vi "VelocityFix.vi"(9 "Tolerance":dbl=1e-05, 10 "Smooth Vel":dbl[][](array[numeric]), 11 "Orig Vel":dbl[][](array[numeric])) -> (3 "Fixed Vel":dbl[][](array[numeric]))   [LabVIEW 2016]
panel:
  out "Array":dbl[](array[numeric])
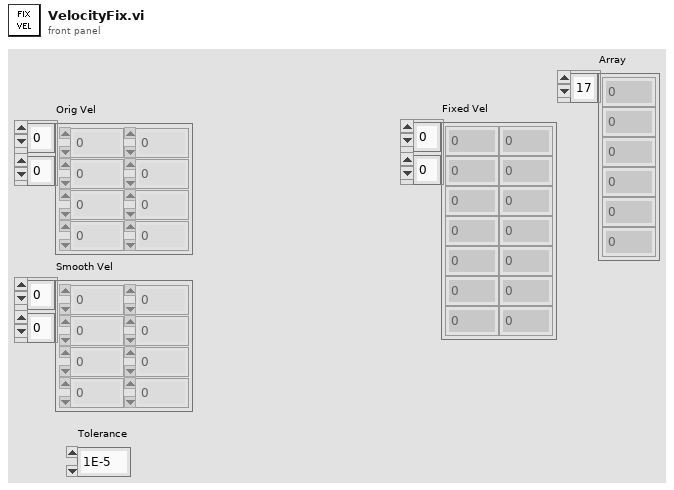
[diagram p1: front panel]
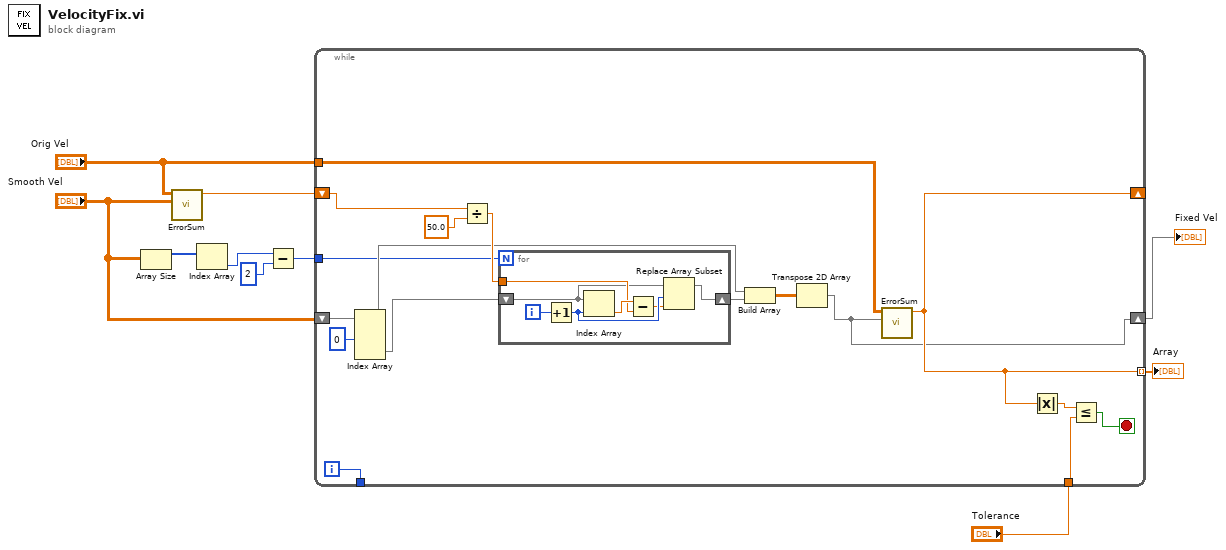
[diagram p0: block diagram]
diagram:
  n1 = Array Size(array="Smooth Vel") -> (size(s)=w3:i32[])
  n2 = call "ErrorSum.vi"("Smooth Vel"="Smooth Vel", "Orig Vel"="Orig Vel") -> ("Difference"=w9:dbl)  [unwired: 9 in]
  n3 = Index Array(array=w3) -> (element=w2:i32)  [unwired: 1 in]
  n4 = Subtract(x=w2, y=2) -> (x-y=w6:i32)
  n5 = while {
    tunnel: "Tolerance" -> [w26]
    tunnel: w6 -> [w12]
    tunnel: "Orig Vel" -> [w21]
    shift-right: [w17] -> _
    shift-left: w9 -> [w19]
    tunnel: [w18] -> _
    tunnel: [w17] -> w5 mode=indexing
    shift-right: [w11] -> w7
    shift-left: "Smooth Vel" -> [w15]
    i -> [w18]
    stop <- w27 stop-if-true
    n6 = Index Array(array=w15, index (col) #1=0 ("disabled index (col)")) -> (element #1=w13:dbl[], element #2=w14:dbl[])  [unwired: 3 in]
    n7 = Divide(x=w19, y=50.0) -> (x/y=w23:dbl)
    n8 = for {
      N: w12 -> [_]
      tunnel: w23 -> [w32]
      shift-right: [w28] -> w22
      shift-left: w14 -> [w31]
      i -> [w34]
      n9 = Increment(x=w34) -> (x+1=w30:i32)
      n10 = Index Array(array=w31, index=w30) -> (element=w33:dbl)
      n11 = Subtract(x=w33, y=w32) -> (x-y=w29:dbl)
      n12 = Replace Array Subset(array=w31, new element=w29, index=w30) -> (w28:dbl[])
    }
    n13 = Build Array(w13, w22) -> (w20:dbl[][])
    n14 = Transpose 2D Array(2D array=w20) -> (transposed array=w11:dbl[][])
    n15 = call "ErrorSum.vi"("Smooth Vel"=w11, "Orig Vel"=w21) -> ("Difference"=w17:dbl)  [unwired: 9 in]
    n16 = Absolute Value(x=w17) -> (abs(x)=w25:dbl)
    n17 = Less Or Equal?(x=w25, y=w26) -> (x <= y?=w27:bool)
  }
  "Fixed Vel" <- w7
  "Array" <- w5
